vi "Edit_BSA_setup.vi"(1 "BSA info":T1={"GPIB Address"="13", "No of Check Bytes"=4, "Extra Info"="57N11", "COLOUR"=52224, "Wavelength (nm)"=52224.0} {"Wavelength (nm)" format="%.1f"}, 3 "BSA 1?":bool, 7 "Multiply Velocity by -1":bool) -> (4 "Centre frequency":dbl format="%.2f", 5 "Bandwidth":dbl format="%.2f", 6 "Output":T5={"Output data format"=enum."Velocity", "Non-validated signals"=enum."Reject"}, 9 "Calibration factor":dbl=3.97 format="%.4f", 10 "Signal conditioning (out)":T6={"High voltage"=2000, "Signal gain (dB)"=45} {"Signal gain (dB)" min=0 max=57 step=1; "High voltage" min=0 max=2040 step=8}, 11 "Buffer mode out":enum16{"One shot", "Ring", "FIFO"}(ring), 12 "Anode current limit (mA)":T8(ring), 14 "Range (out)":T7={"Centre frequency"=16, "Bandwidth"=10, "Units"=enum."m/s", "Frequency shift"=enum."Enabled"} {"Bandwidth" items=["3.776E-3", "7.553E-3", "15.105E-3", "30.211E-3", "60.422E-3", "120.844E-3", "241.687E-3", "483.375E-3", "966.750E-3", "1.933E+0", "3.867E+0", "7.734E+0", "15.468E+0", "30.936E+0"]; "Centre frequency" items=["-15.468E+0", "-14.501E+0", "-13.534E+0", "-12.568E+0", "-11.601E+0", "-10.634E+0", "-9.667E+0", "-8.701E+0", "-7.734E+0", "-6.767E+0", "-5.800E+0", "-4.834E+0", "-3.867E+0", "-2.900E+0", "-1.933E+0", "-966.750E-3", "0.000E+0", "966.750E-3", "1.933E+0", "2.900E+0", "3.867E+0", "4.834E+0", "5.800E+0", "6.767E+0", "7.734E+0", "8.701E+0", "9.667E+0", "10.634E+0", "11.601E+0", "12.568E+0", "13.534E+0", "14.501E+0", "15.468E+0"]}, 15 "Selected range":cluster{"Minimum":dbl, "Maximum":dbl}={"Minimum"=-1.9850000000000005, "Maximum"=1.9850000000000005} {"Maximum" format="%.2f"; "Minimum" format="%.2f"}, 17 "Clock parameters (out)":T2={"Arrival time clock"=enum."Internal", "Clock source"=enum."Private", "Coincidence"=enum."Master"}, 18 "Data collection mode (out)":T4 {"Duty cycle (%)" format="%.2f"; "Dead time (s)" format="%.2f"}, 19 "Analysis parameters (out)":T3={"Burst criterion"=enum."Envelope", "Oversize reject level"=enum."1 (disabled)", "Pedestal attenuation"=enum."0", "Record length"=enum."16", "Quality factor"=0} {"Quality factor" min=0 max=80 step=10})   [LabVIEW 2010]
uses:
  Controls/ok_button.ctl
  Controls/BSA_info_Cluster.ctl
  Globals/LDA_meas_global_1.vi
  Globals/LDA_meas_global_2.vi
panel:
  out "45 Degree Mirror":bool
  out "Probe Configuration":string
  in  "Component":string="W"
  out "error out":errorcluster
  in  "Clock parameters":T2={"Arrival time clock"=enum."Internal", "Clock source"=enum."Private", "Coincidence"=enum."Master"}
  in  "Analysis parameters":T3={"Burst criterion"=enum."Envelope", "Oversize reject level"=enum."1 (disabled)", "Pedestal attenuation"=enum."0", "Record length"=enum."16", "Quality factor"=0} {"Quality factor" min=0 max=80 step=10}
  in  "Data collection mode":T4 {"Duty cycle (%)" format="%.2f"; "Dead time (s)" format="%.2f"}
  in  "Buffer mode":enum16{"One shot", "Ring", "FIFO"}(ring)
  in  "OK":T9
  in  "Signal conditioning":T6={"High voltage"=1600, "Signal gain (dB)"=35} {"Signal gain (dB)" min=0 max=57 step=1; "High voltage" min=0 max=1600 step=8}
  in  "Range":T10={"Centre Velocity"=16, "Velocity span"=10, "Units"=enum."m/s", "Frequency shift"=enum."Enabled"} {"Velocity span" items=["3.582E-3", "7.164E-3", "14.328E-3", "28.656E-3", "57.312E-3", "114.625E-3", "229.250E-3", "458.500E-3", "917.000E-3", "1.834E+0", "3.668E+0", "7.336E+0", "14.672E+0", "29.344E+0"]; "Centre Velocity" items=["-7.336E+0", "-6.877E+0", "-6.419E+0", "-5.960E+0", "-5.502E+0", "-5.043E+0", "-4.585E+0", "-4.127E+0", "-3.668E+0", "-3.209E+0", "-2.751E+0", "-2.292E+0", "-1.834E+0", "-1.375E+0", "-917.000E-3", "-458.500E-3", "0.000E+0", "458.500E-3", "917.000E-3", "1.375E+0", "1.834E+0", "2.292E+0", "2.751E+0", "3.209E+0", "3.668E+0", "4.127E+0", "4.585E+0", "5.043E+0", "5.502E+0", "5.960E+0", "6.419E+0", "6.877E+0", "7.336E+0"]}
  # "These values can be\nchanged in LDA Setup\nrun from the EnFlo Hub"
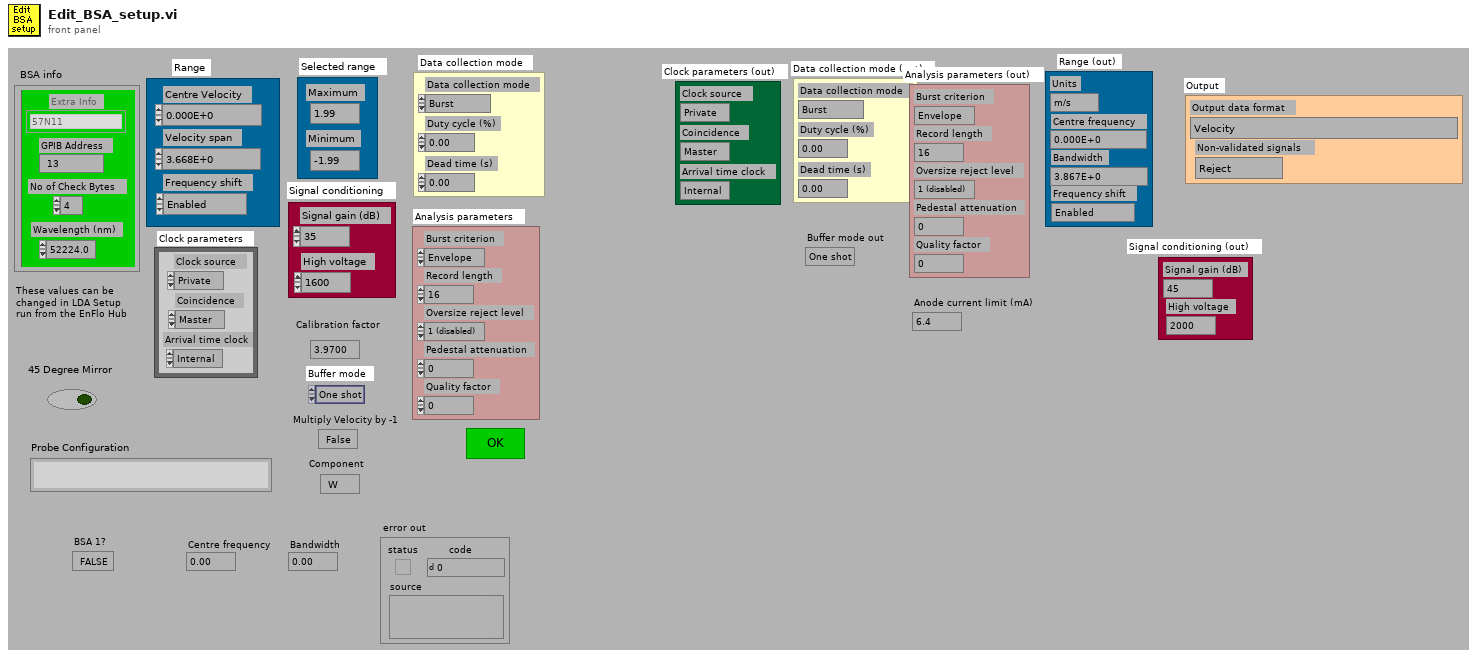
[diagram p1: front panel]
types:
  T1 = typedef "BSA_info_Cluster.ctl" = cluster{"GPIB Address":string, "No of Check Bytes":i32, "Extra Info":string, "COLOUR":u32, "Wavelength (nm)":dbl}
  T2 = cluster{"Arrival time clock":enum16{"External", "Internal"}, "Clock source":enum16{"Slave", "Master", "Private"}, "Coincidence":enum16{"Slave", "Master", "Private"}}
  T3 = cluster{"Burst criterion":enum16{"Envelope", "Pedestal", "Env and ped"}, "Oversize reject level":enum16{"1 (disabled)", "2", "3", "4", "5", "6", "7", "8", "9"}, "Pedestal attenuation":enum16{"0", "6", "12", "18"}, "Record length":enum16{"8", "16", "32", "64"}, "Quality factor":i16}
  T4 = cluster{"Dead time (s)":dbl, "Duty cycle (%)":dbl, "Data collection mode":enum16{"Burst", "Contiuous", "Dead time", "External"}}
  T5 = cluster{"Output data format":enum16{"Velocity, transit time, arrival time", "Velocity, arrival time", "Velocity, transit time", "Velocity"}, "Non-validated signals":enum16{"Accept", "Reject"}}
  T6 = cluster{"High voltage":i16, "Signal gain (dB)":i16}
  T7 = cluster{"Centre frequency":u16, "Bandwidth":u16, "Units":enum16{"Hz", "m/s"}, "Frequency shift":enum16{"Disabled", "Enabled"}}
  T8 = enum16{"6.4", "3.2", "1.6", "0.8", "0.4", "0.2", "0.1", "0.05"}
  T9 = typedef "ok_button.ctl" = bool
  T10 = cluster{"Centre Velocity":u16, "Velocity span":u16, "Units":enum16{"Hz", "m/s"}, "Frequency shift":enum16{"Disabled", "Enabled"}}
  T11 = enum16{"Burst", "Contiuous", "Dead time", "External"}
  T12 = enum16{"1 (disabled)", "2", "3", "4", "5", "6", "7", "8", "9"}
  T13 = enum16{"Velocity, transit time, arrival time", "Velocity, arrival time", "Velocity, transit time", "Velocity"}
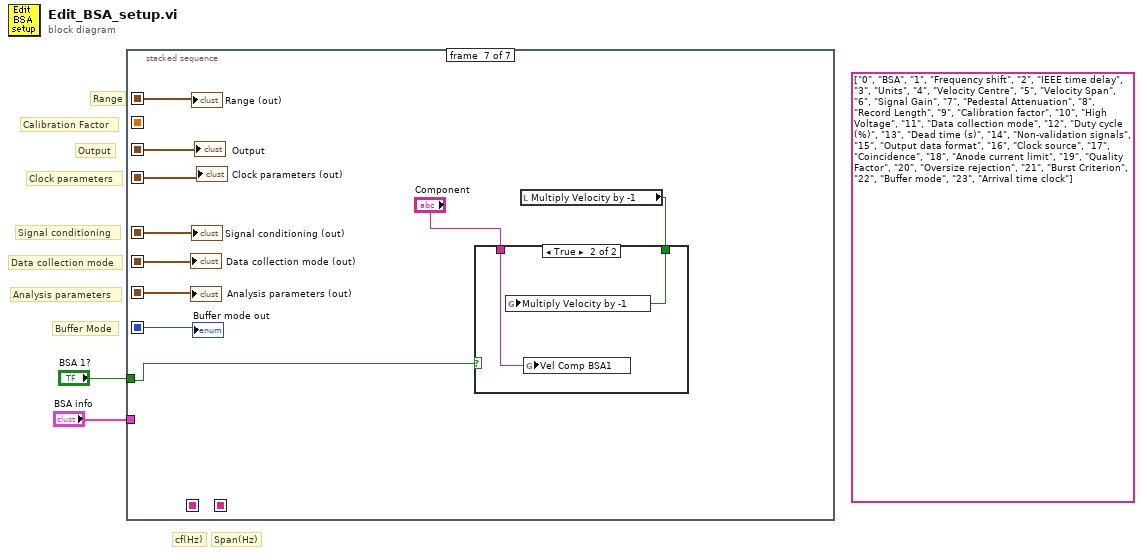
[diagram p0: block diagram]
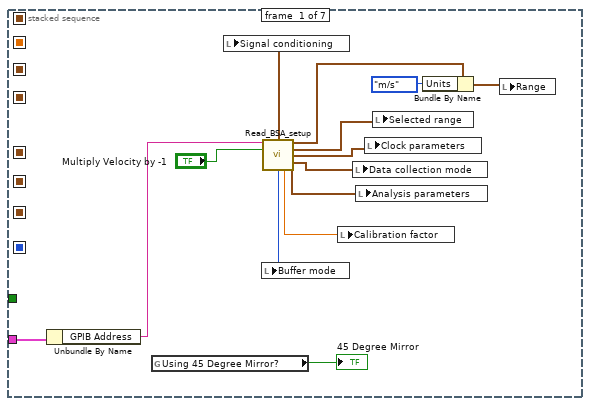
[diagram p2: hidden frame]
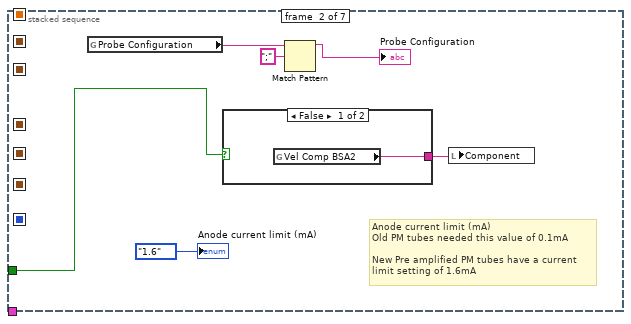
[diagram p3: hidden frame]
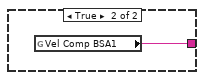
[diagram p4: hidden frame]
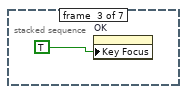
[diagram p5: hidden frame]
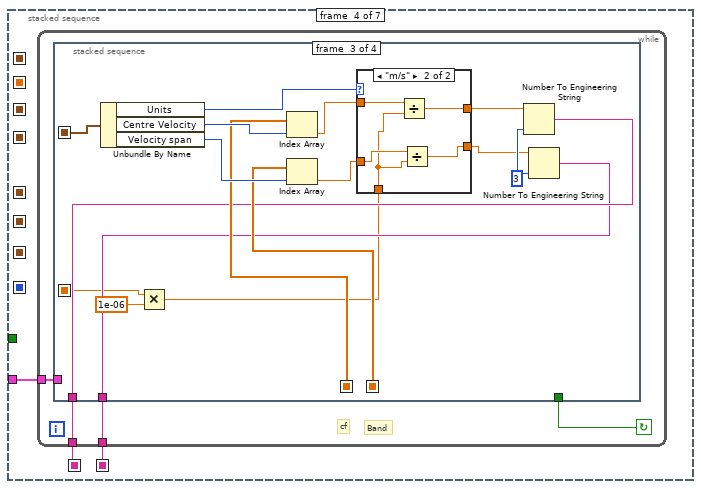
[diagram p6: hidden frame]
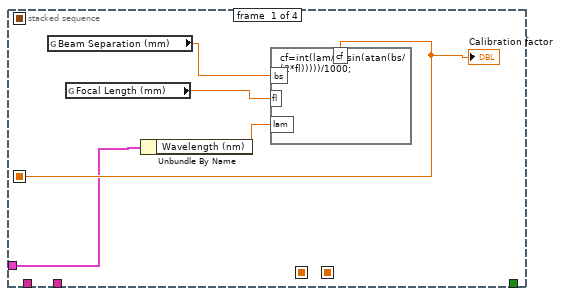
[diagram p7: hidden frame]
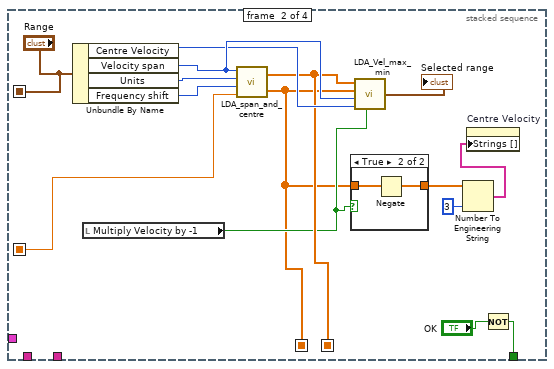
[diagram p8: hidden frame]
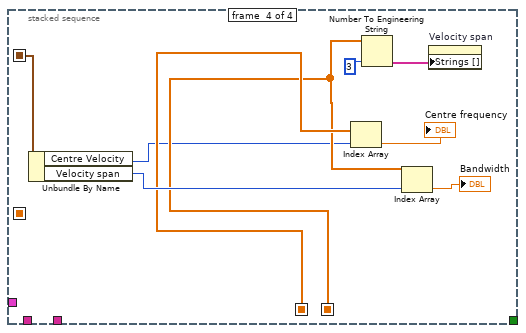
[diagram p11: hidden frame]
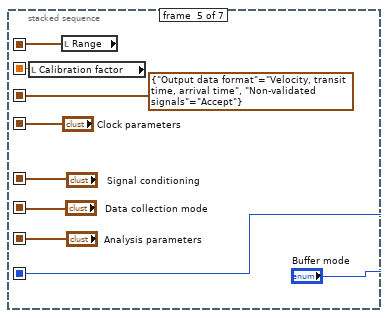
[diagram p12: hidden frame]
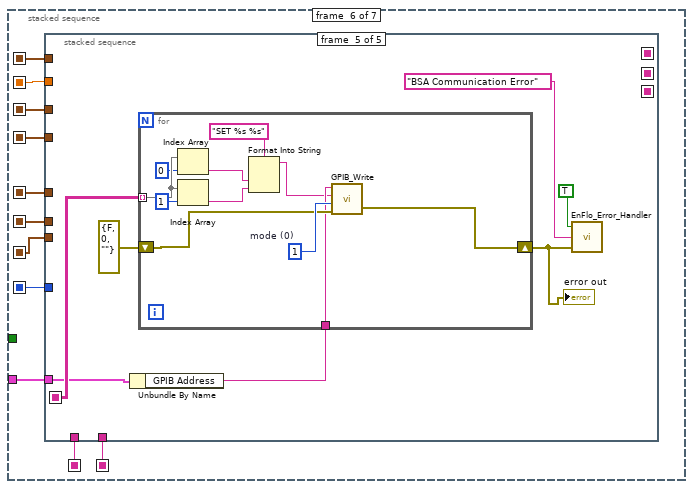
[diagram p13: hidden frame]
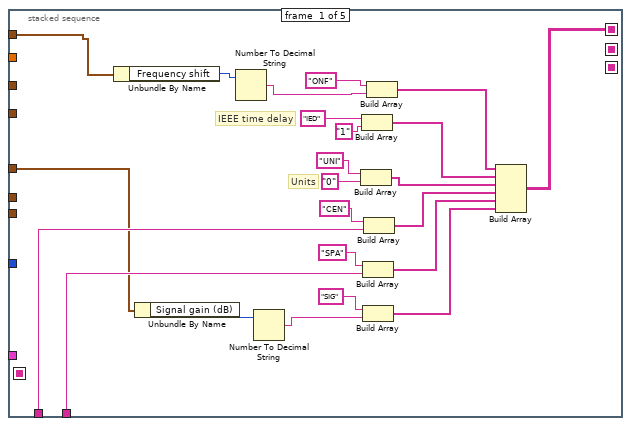
[diagram p14: hidden frame]
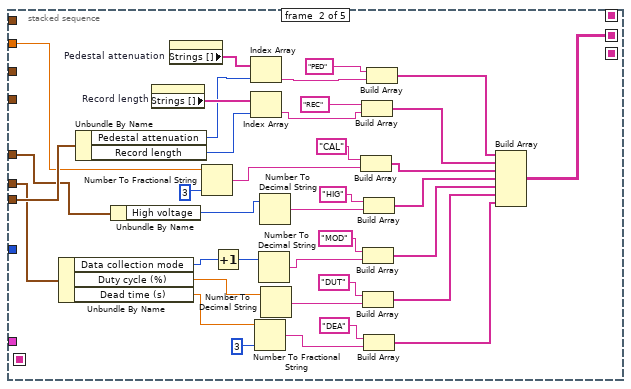
[diagram p15: hidden frame]
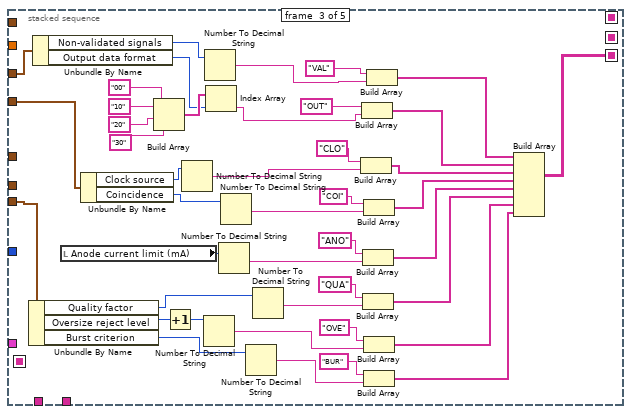
[diagram p16: hidden frame]
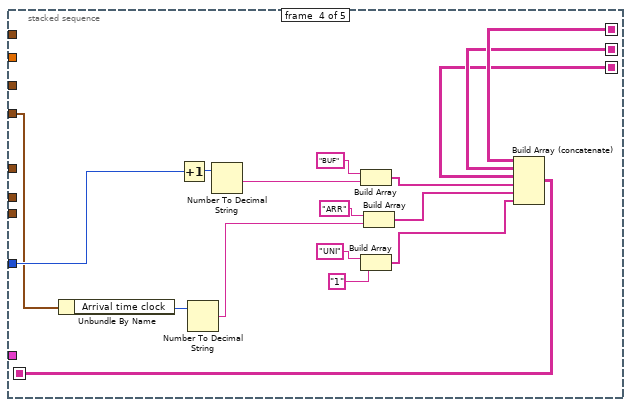
[diagram p17: hidden frame]
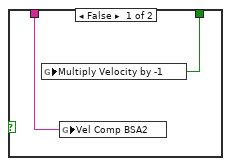
[diagram p18: hidden frame]
diagram:
  (unwired) string[][] [["0", "BSA"], ["1", "Frequency shift"], ["2", "IEEE time delay"], ["3", "Units"], ["4", "Velocity Centre"], ["5", "Velocity Span"], ["6", "Signal Gain"], ["7", "Pedestal Attenuation"], ["8", "Record Length"], ["9", "Calibration factor"], ["10", "High Voltage"], ["11", "Data collection mode"], ["12", "Duty cycle (%)"], ["13", "Dead time (s)"], ["14", "Non-validation signals"], ["15", "Output data format"], ["16", "Clock source"], ["17", "Coincidence"], ["18", "Anode current limit"], ["19", "Quality Factor"], ["20", "Oversize rejection"], ["21", "Burst Criterion"], ["22", "Buffer mode"], ["23", "Arrival time clock"]]
  # "Span(Hz)"
  # "cf(Hz)"
  # "Buffer Mode"
  # "Clock parameters"
  # "Output"
  # "Calibration Factor"
  # "Data collection mode"
  # "Analysis parameters"
  # "Signal conditioning"
  # "Range"
  n1 = stacked-sequence {
    seq-local: [_ _ _ _ w92 _ _] -> [_ _ _ _ _ w106 w253]
    seq-local: [_ _ _ _ w93 _ _] -> [_ _ _ _ _ w101 _]
    seq-local: [_ _ _ _ T5 {"Output data format"=enum."Velocity, transit time, arrival time", "Non-validated signals"=enum."Accept"} ("Output") _ _] -> [_ _ _ _ _ w99 w248]
    seq-local: [_ _ _ _ "Clock parameters" _ _] -> [_ _ _ _ _ w98 w249]
    seq-local: [_ _ _ _ "Signal conditioning" _ _] -> [_ _ _ _ _ w103 w250]
    seq-local: [_ _ _ _ "Data collection mode" _ _] -> [_ _ _ _ _ w100 w252]
    seq-local: [_ _ _ _ "Analysis parameters" _ _] -> [_ _ _ _ _ w102 w251]
    seq-local: [_ _ _ _ "Buffer mode" _ _] -> [_ _ _ _ _ w97 w244]
    seq-local: [_ _ _ w28 _ _ _] -> [_ _ _ _ _ w105 _]
    seq-local: [_ _ _ w27 _ _ _] -> [_ _ _ _ _ w104 _]
    tunnel: "BSA 1?" -> [_ w20 _ _ _ _ w247]
    tunnel: "BSA info" -> [w5 _ _ w26 _ w96 _]
    frame #0 {
      n2 = Unbundle By Name(w5) -> ("GPIB Address"=w4:string)
      n3 = global read "LDA_meas_global_1.vi" "Using 45 Degree Mirror?"() -> (→"45 Degree Mirror":bool)
      n4 = call "Read_BSA_setup.vi"("GPIB Address"=w4, "Multiply Velocity by -1"="Multiply Velocity by -1") -> ("Signal conditioning"=w16:T6, "Range"=w9:T10, "Selected range"=w10:cluster{"Minimum":dbl, "Maximum":dbl}, "Clock parameters"=w11:T2, "Data collection mode"=w12:T4, "Buffer mode"=w15:enum16{"One shot", "Ring", "FIFO"}, "Calibration factor"=w14:dbl, "Analysis parameters"=w13:T3)  [unwired: 1 in, 5 out]
      n5 = local write "Signal conditioning"(w16) -> ()
      n6 = local write "Buffer mode"(w15) -> ()
      n7 = local write "Calibration factor"(w14) -> ()
      n8 = local write "Data collection mode"(w12) -> ()
      n9 = local write "Analysis parameters"(w13) -> ()
      n10 = local write "Clock parameters"(w11) -> ()
      n11 = local write "Selected range"(w10) -> ()
      n12 = Bundle By Name(cluster=w9, "Units"=enum16{"Hz", "m/s"}."m/s") -> (w8:T10)
      n13 = local write "Range"(w8) -> ()
    }
    frame #1 {
      # "Anode current limit (mA)\nOld PM tubes needed this value of 0.1mA\n\nNew Pre amplified PM tubes have a current\nlimit setting of 1.6mA"
      n14 = global read "LDA_meas_global_1.vi" "Probe Configuration"() -> (w19:string)
      n15 = case shown="False" w20 {
        tunnel: [w23 w24] -> w21
        frame False {
          n16 = global read "LDA_meas_global_2.vi" "Vel Comp BSA2"() -> (w23:string)
        }
        frame True {
          n17 = global read "LDA_meas_global_1.vi" "Vel Comp BSA1"() -> (w24:string)
        }
      }
      n18 = Match Pattern(string=w19, regular expression=";") -> (before substring=→"Probe Configuration":string)  [unwired: 4 out]
      n19 = local write "Component"(w21) -> ()
      "Anode current limit (mA)" <- T8."1.6" ("Anode current limit (mA)")
    }
    frame #2 {
      n20 = property on="OK" class="Bool"("Key Focus"=TRUE ("Visible")) -> ()  [unwired: 2 in, 2 out]
    }
    frame #3 {
      n21 = while {
        tunnel: [w30] -> w27
        tunnel: [w31] -> w28
        tunnel: w26 -> [w29]
        stop <- w32 continue-if-true
        # "Band"
        # "cf"
        n22 = stacked-sequence {
          seq-local: [w34 _ _ _] -> [_ w38 w63 _]
          seq-local: [_ w39 _ _] -> [_ _ w67 w83]
          seq-local: [_ w44 _ _] -> [_ _ w66 w82]
          seq-local: [_ "Range" _ _] -> [_ _ w71 w87]
          tunnel: [_ w51 _ _] -> w32
          tunnel: [_ _ w65 _] -> w31
          tunnel: [_ _ w64 _] -> w30
          tunnel: w29 -> [w33 _ _ _]
          frame #0 {
            n23 = global read "LDA_meas_global_1.vi" "Beam Separation (mm)"() -> (w36:dbl)
            n24 = global read "LDA_meas_global_1.vi" "Focal Length (mm)"() -> (w35:dbl)
            n25 = Unbundle By Name(w33) -> ("Wavelength (nm)"=w37:dbl)
            n26 = formula code="cf=int(lam/2/(sin(atan(bs/(2*fl)))))/1000;"("bs"=w36, "fl"=w35, "lam"=w37) -> ("cf"=w34:dbl)
            "Calibration factor" <- w34
          }
          frame #1 {
            n27 = Unbundle By Name("Range") -> ("Centre Velocity"=w46:u16, "Velocity span"=w47:u16, "Units"=w49:enum16{"Hz", "m/s"}, "Frequency shift"=w48:enum16{"Disabled", "Enabled"})
            n28 = local read "Multiply Velocity by -1"() -> (w43:bool)
            n29 = call "LDA_span_and_centre.vi"("Calibration factor"=w38, "Frequency shift"=w48, "Units"=w49, "Velocity span"=w47) -> ("Centres"=w39:dbl[], "Spans"=w44:dbl[])
            n30 = case shown="True" w43 {
              tunnel: [w53 w54] -> w40
              tunnel: w39 -> [w53 w55]
              frame False {
              }
              frame True {
                n31 = Negate(x=w55) -> (-x=w54:dbl[])
              }
            }
            n32 = call "LDA_Vel_max_min.vi"("Multiply Velocity by -1"=w43, "Centre Velocity"=w46, "Velocity span"=w47, "Centres"=w39, "Spans"=w44) -> ("Selected range"=→"Selected range":cluster{"Minimum":dbl, "Maximum":dbl})  [unwired: 1 out]
            n33 = Number To Engineering String(2:i16 3 ("precision (6)"), 4:w40) -> (0:w41:string[])  [unwired: 2 out]
            n34 = property on="Centre Velocity" class="Ring (strict)"("Strings []"=w41) -> ()  [unwired: 2 in, 2 out]
            n35 = Not(x="OK") -> (.not. x?=w51:T9)
          }
          frame #2 {
            w68 = 3
            n36 = Unbundle By Name(w71) -> ("Units"=w58:enum16{"Hz", "m/s"}, "Centre Velocity"=w69:u16, "Velocity span"=w70:u16)
            n37 = Multiply(x=w63, y=1e-06) -> (x*y=w61:dbl)
            n38 = Index Array(array=w67, index=w69) -> (element=w59:dbl)
            n39 = Index Array(array=w66, index=w70) -> (element=w60:dbl)
            n40 = case shown="\"m/s\"" w58 {
              tunnel: w59 -> [w73 w78]
              tunnel: [w73 w74] -> w57
              tunnel: w60 -> [w72 w77]
              tunnel: [w72 w75] -> w56
              tunnel: w61 -> [_ w76]
              frame "Hz" {
              }
              frame "m/s" {
                n41 = Divide(x=w78, y=w76) -> (x/y=w74:dbl)
                n42 = Divide(x=w77, y=w76) -> (x/y=w75:dbl)
              }
            }
            n43 = Number To Engineering String(2:w68, 4:w57) -> (0:w65:string)  [unwired: 2 out]
            n44 = Number To Engineering String(2:w68, 4:w56) -> (0:w64:string)  [unwired: 2 out]
          }
          frame #3 {
            n45 = Unbundle By Name(w87) -> ("Centre Velocity"=w80:u16, "Velocity span"=w84:u16)
            n46 = Index Array(array=w83, index=w80) -> (element=→"Centre frequency":dbl)
            n47 = Number To Engineering String(2:3, 4:w82) -> (0:w81:string[])  [unwired: 2 out]
            n48 = Index Array(array=w82, index=w84) -> (element=→"Bandwidth":dbl)
            n49 = property on="Velocity span" class="Ring (strict)"("Strings []"=w81) -> ()  [unwired: 2 in, 2 out]
          }
        }
      }
    }
    frame #4 {
      n50 = local read "Calibration factor"() -> (w93:dbl)
      n51 = local read "Range"() -> (w92:T10)
    }
    frame #5 {
      n52 = stacked-sequence {
        seq-local: [w107 _ _ _ _] -> [_ _ _ w215 _]
        seq-local: [_ w130 _ _ _] -> [_ _ _ w214 _]
        seq-local: [_ _ w167 _ _] -> [_ _ _ w213 _]
        seq-local: [_ _ _ w212 _] -> [_ _ _ _ w232]
        tunnel: w106 -> [w129 _ _ _ _]
        tunnel: w105 -> [w120 _ _ _ _]
        tunnel: w104 -> [w118 _ _ _ _]
        tunnel: w103 -> [w115 w144 _ _ _]
        tunnel: w102 -> [_ w152 w176 _ _]
        tunnel: w101 -> [_ w146 _ _ _]
        tunnel: w100 -> [_ w141 _ _ _]
        tunnel: w99 -> [_ _ w194 _ _]
        tunnel: w98 -> [_ _ w184 w218 _]
        tunnel: w97 -> [_ _ _ w220 _]
        tunnel: w96 -> [_ _ _ _ w228]
        frame #0 {
          # "Units"
          # "IEEE time delay"
          n53 = Unbundle By Name(w129) -> ("Frequency shift"=w128:enum16{"Disabled", "Enabled"})
          n54 = Unbundle By Name(w115) -> ("Signal gain (dB)"=w116:i16)
          n55 = Number To Decimal String(number=w128) -> (decimal integer string=w126:string)  [unwired: 1 out]
          n56 = Number To Decimal String(number=w116) -> (decimal integer string=w114:string)  [unwired: 1 out]
          n57 = Build Array("UNI", "0") -> (w111:string[])
          n58 = Build Array("IED", "1" ("element")) -> (w112:string[])
          n59 = Build Array("SPA", w118) -> (w109:string[])
          n60 = Build Array("SIG", w114) -> (w108:string[])
          n61 = Build Array("CEN", w120) -> (w110:string[])
          n62 = Build Array("ONF", w126) -> (w113:string[])
          n63 = Build Array(w113, w112, w111, w110, w109, w108) -> (w107:string[][])
        }
        frame #1 {
          n64 = Unbundle By Name(w141) -> ("Data collection mode"=w136:T11, "Duty cycle (%)"=w135:dbl, "Dead time (s)"=w134:dbl)
          n65 = Unbundle By Name(w152) -> ("Pedestal attenuation"=w151:enum16{"0", "6", "12", "18"}, "Record length"=w150:enum16{"8", "16", "32", "64"})
          n66 = Unbundle By Name(w144) -> ("High voltage"=w143:i16)
          n67 = property on="Record length" class="Enum (strict)"() -> ("Strings []"=w153:string[])  [unwired: 2 in, 2 out]
          n68 = property on="Pedestal attenuation" class="Enum (strict)"() -> ("Strings []"=w154:string[])  [unwired: 2 in, 2 out]
          n69 = Number To Fractional String(number=w146, precision (6)=3) -> (F-format string=w145:string)  [unwired: 2 out]
          n70 = Increment(x=w136) -> (x+1=w139:T11)
          n71 = Index Array(array=w154, index=w151) -> (element=w148:string)
          n72 = Index Array(array=w153, index=w150) -> (element=w149:string)
          n73 = Number To Fractional String(number=w134, precision (6)=3) -> (F-format string=w133:string)  [unwired: 2 out]
          n74 = Number To Decimal String(number=w139) -> (decimal integer string=w131:string)  [unwired: 1 out]
          n75 = Number To Decimal String(number=w143) -> (decimal integer string=w142:string)  [unwired: 1 out]
          n76 = Number To Decimal String(number=w135) -> (decimal integer string=w132:string)  [unwired: 1 out]
          n77 = Build Array("CAL", w145) -> (w158:string[])
          n78 = Build Array("REC", w149) -> (w159:string[])
          n79 = Build Array("MOD", w131) -> (w156:string[])
          n80 = Build Array("DUT", w132) -> (w155:string[])
          n81 = Build Array("HIG", w142) -> (w157:string[])
          n82 = Build Array("DEA", w133) -> (w137:string[])
          n83 = Build Array("PED", w148) -> (w160:string[])
          n84 = Build Array(w160, w159, w158, w157, w156, w155, w137) -> (w130:string[][])
        }
        frame #2 {
          n85 = Unbundle By Name(w176) -> ("Quality factor"=w174:i16, "Oversize reject level"=w173:T12, "Burst criterion"=w172:enum16{"Envelope", "Pedestal", "Env and ped"})
          n86 = Unbundle By Name(w194) -> ("Non-validated signals"=w188:enum16{"Accept", "Reject"}, "Output data format"=w187:T13)
          n87 = local read "Anode current limit (mA)"() -> (w179:T8)
          n88 = Unbundle By Name(w184) -> ("Clock source"=w183:enum16{"Slave", "Master", "Private"}, "Coincidence"=w182:enum16{"Slave", "Master", "Private"})
          n89 = Build Array("00", "10", "20", "30") -> (w189:string[])
          n90 = Increment(x=w173) -> (x+1=w175:T12)
          n91 = Number To Decimal String(number=w183) -> (decimal integer string=w181:string)  [unwired: 1 out]
          n92 = Number To Decimal String(number=w175) -> (decimal integer string=w170:string)  [unwired: 1 out]
          n93 = Number To Decimal String(number=w188) -> (decimal integer string=w186:string)  [unwired: 1 out]
          n94 = Index Array(array=w189, index=w187) -> (element=w185:string)
          n95 = Number To Decimal String(number=w179) -> (decimal integer string=w178:string)  [unwired: 1 out]
          n96 = Number To Decimal String(number=w182) -> (decimal integer string=w180:string)  [unwired: 1 out]
          n97 = Number To Decimal String(number=w172) -> (decimal integer string=w171:string)  [unwired: 1 out]
          n98 = Number To Decimal String(number=w174) -> (decimal integer string=w169:string)  [unwired: 1 out]
          n99 = Build Array("CLO", w181) -> (w200:string[])
          n100 = Build Array("OUT", w185) -> (w201:string[])
          n101 = Build Array("ANO", w178) -> (w198:string[])
          n102 = Build Array("QUA", w169) -> (w197:string[])
          n103 = Build Array("COI", w180) -> (w199:string[])
          n104 = Build Array("OVE", w170) -> (w195:string[])
          n105 = Build Array("BUR", w171) -> (w168:string[])
          n106 = Build Array("VAL", w186) -> (w202:string[])
          n107 = Build Array(w202, w201, w200, w199, w198, w197, w195, w168) -> (w167:string[][])
        }
        frame #3 {
          n108 = Unbundle By Name(w218) -> ("Arrival time clock"=w217:enum16{"External", "Internal"})
          n109 = Increment(x=w220) -> (x+1=w221:enum16{"One shot", "Ring", "FIFO"})
          n110 = Number To Decimal String(number=w217) -> (decimal integer string=w216:string)  [unwired: 1 out]
          n111 = Number To Decimal String(number=w221) -> (decimal integer string=w219:string)  [unwired: 1 out]
          n112 = Build Array("BUF", w219) -> (w223:string[])
          n113 = Build Array("UNI", "1" ("element")) -> (w209:string[])
          n114 = Build Array("ARR", w216) -> (w222:string[])
          n115 = Build Array (concatenate)(w215, w214, w213, w223, w222, w209) -> (w212:string[][])
        }
        frame #4 {
          n116 = Unbundle By Name(w228) -> ("GPIB Address"=w227:string)
          n117 = for {
            tunnel: w232 -> [w239] mode=indexing
            shift-right: [w242] -> w226
            shift-left: errorcluster {"status"=FALSE, "code"=0, "source"=""} ("error out") -> [w241]
            tunnel: w227 -> [w240]
            w243 = i16 1  # mode (0)
            n118 = Index Array(array=w239, index=0) -> (element=w236:string)
            n119 = Index Array(array=w239, index=1) -> (element=w235:string)
            n120 = Format Into String(format string="SET %s %s", w236, w235) -> (resulting string=w233:string)  [unwired: 2 in, 1 out]
            n121 = call "GPIB_Write.vi"("address string"=w240, "data In"=w233, "mode (0)"=w243, "error in"=w241) -> ("error out"=w242:errorcluster)  [unwired: 1 in, 1 out]
          }
          "error out" <- w226
          n122 = call "EnFlo_Error_Handler.vi"("error in (no error)"=w226, "Error Type"="BSA Communication Error", "Dialog Box (T)"=TRUE) -> ()  [unwired: 3 out]
        }
      }
    }
    frame #6 {
      n123 = local read "Multiply Velocity by -1"() -> (w245:bool)
      n124 = case shown="True" w247 {
        tunnel: "Component" -> [w255 w257]
        tunnel: w245 -> [w254 w256]
        frame False {
          n125 = global write "LDA_meas_global_2.vi" "Multiply Velocity by -1"(w254) -> ()
          n126 = global write "LDA_meas_global_2.vi" "Vel Comp BSA2"(w255) -> ()
        }
        frame True {
          n127 = global write "LDA_meas_global_1.vi" "Multiply Velocity by -1"(w256) -> ()
          n128 = global write "LDA_meas_global_1.vi" "Vel Comp BSA1"(w257) -> ()
        }
      }
      "Range (out)" <- w253
      "Signal conditioning (out)" <- w250
      "Analysis parameters (out)" <- w251
      "Output" <- w248
      "Clock parameters (out)" <- w249
      "Data collection mode (out)" <- w252
      "Buffer mode out" <- w244
    }
  }
